vi "Config Math.vi"(0 "VISA resource name":refnum<visa-resource-name>, 1 "Linear Variable M (0.0000)":dbl min=-9999.9 max=9999.9 step=0.0001 format="%.4f", 2 "Linear Variable B (0.0000)":dbl min=-9999.9 max=9999.9 step=0.0001 format="%.4f", 3 "Linear X Source (0:Kelvin)":u16(ring) items=["Kelvin", "Celsius", "Sensor Units"], 5 "Input (1)":dbl=1.0 min=1.0 max=8.0 step=1.0, 7 "Min/Max Source (0:Kelvin)":u16(ring) items=["Kelvin", "Celsius", "Sensor Units", "Linear Data"], 9 "Filter (F: Filter OFF)":bool, 11 "error in (no error)":errorcluster, 12 "Filter Points (8)":dbl=8.0 min=2.0 max=64.0 step=1.0, 13 "Filter Window (8)":dbl=8.0 min=1.0 max=10.0 step=1.0) -> (4 "VISA resource name out":refnum<visa-resource-name>, 15 "error out":errorcluster)   [LabVIEW 2012, in "Lake Shore Cryotronics 218.lvlib"]
doc: "This VI configures all math functions for the selected input. Math functions include min/max source, filter settings, and linear equation parameters."
uses:
  <instrlib>/Lake Shore Cryotronics 218/Lake Shore Cryotronics 218.lvlib
panel:
  # "Filter ON\nFilter OFF"
  # "%"
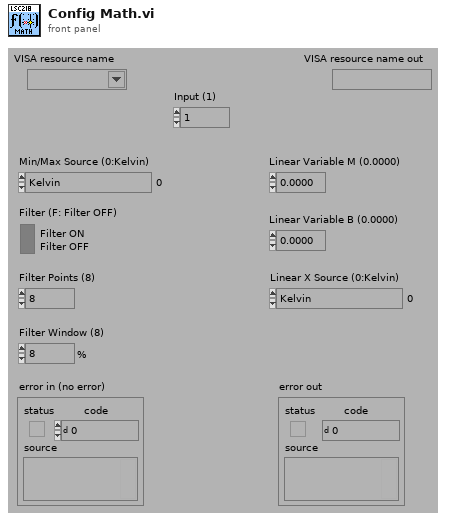
[diagram p1: front panel]
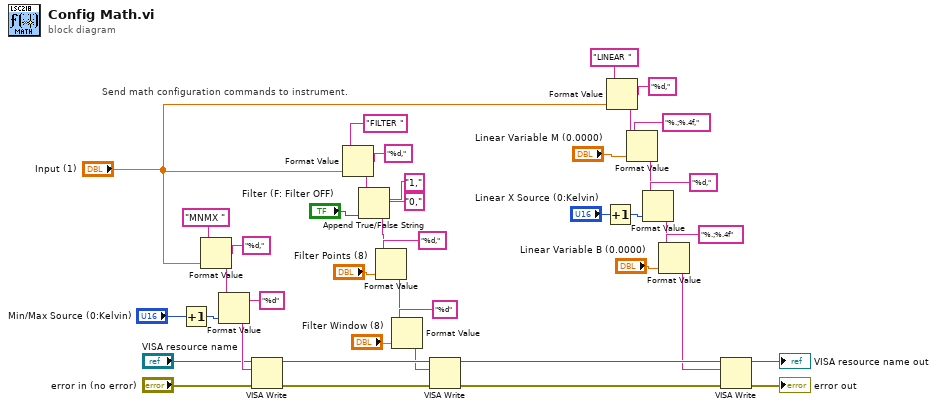
[diagram p0: block diagram]
diagram:
  # "Send math configuration commands to instrument."
  n1 = Increment(x="Min/Max Source (0:Kelvin)") -> (x+1=w5:u16)
  n2 = Format Value(string ("")="MNMX ", format string="%d,", value (0)="Input (1)") -> (output string=w26:string)
  n3 = Format Value(string ("")=w26, format string="%d", value (0)=w5) -> (output string=w38:string)
  n4 = VISA Write(VISA resource name="VISA resource name", write buffer=w38, error in (no error)="error in (no error)") -> (VISA resource name out=w37:refnum<visa-resource-name>, error out=w36:errorcluster)  [unwired: 1 out]
  n5 = Format Value(string ("")="FILTER ", format string="%d,", value (0)="Input (1)") -> (output string=w31:string)
  n6 = Append True/False String(1:"Filter (F: Filter OFF)", 2:"0,", 3:"1,", 4:w31) -> (0:w21:string)
  n7 = Format Value(string ("")=w21, format string="%d,", value (0)="Filter Points (8)") -> (output string=w20:string)
  n8 = Format Value(string ("")=w20, format string="%d", value (0)="Filter Window (8)") -> (output string=w19:string)
  n9 = VISA Write(VISA resource name=w37, write buffer=w19, error in (no error)=w36) -> (VISA resource name out=w34:refnum<visa-resource-name>, error out=w35:errorcluster)  [unwired: 1 out]
  n10 = Increment(x="Linear X Source (0:Kelvin)") -> (x+1=w6:u16)
  n11 = Format Value(string ("")="LINEAR ", format string="%d,", value (0)="Input (1)") -> (output string=w28:string)
  n12 = Format Value(string ("")=w28, format string="%.;%.4f,", value (0)="Linear Variable M (0.0000)") -> (output string=w13:string)
  n13 = Format Value(string ("")=w13, format string="%d,", value (0)=w6) -> (output string=w12:string)
  n14 = Format Value(string ("")=w12, format string="%.;%.4f", value (0)="Linear Variable B (0.0000)") -> (output string=w11:string)
  n15 = VISA Write(VISA resource name=w34, write buffer=w11, error in (no error)=w35) -> (VISA resource name out=→"VISA resource name out":refnum<visa-resource-name>, error out=→"error out":errorcluster)  [unwired: 1 out]
